vi "Image Compression with DCT.vi"() -> ()   [LabVIEW 2023]
doc: "This VI uses the DCT VI to compress images. LabVIEW transforms the Source Image to DCT Coefficients in 8-by-8 blocks, then the inverse DCT transforms the image back to Restored Image."
uses:
  <vilib>/Analysis/2dsp.llb/2D DCT.vi
  <vilib>/Analysis/2dsp.llb/2D Inverse DCT.vi
  <vilib>/Analysis/NI_AALPro.lvlib
panel:
  out "Number of block size":i32
  out "Mean Square Error (MSE)":dbl
  in  "Set All":bool
  in  "Clear All":bool
  in  "Truncated Pattern":bool[][](array[boolean])=[[TRUE, TRUE, TRUE, TRUE, FALSE, FALSE, FALSE, FALSE], [TRUE, TRUE, TRUE, FALSE, FALSE, FALSE, FALSE, FALSE], [TRUE, TRUE, FALSE, FALSE, FALSE, FALSE, FALSE, FALSE], [TRUE, FALSE, FALSE, FALSE, FALSE, FALSE, FALSE, FALSE], [FALSE, FALSE, FALSE, FALSE, FALSE, FALSE, FALSE, FALSE], [FALSE, FALSE, FALSE, FALSE, FALSE, FALSE, FALSE, FALSE], [FALSE, FALSE, FALSE, FALSE, FALSE, FALSE, FALSE, FALSE], [FALSE, FALSE, FALSE, FALSE, FALSE, FALSE, FALSE, FALSE]]
  in  "Stop":bool
  out "Restored Image":u8[][](graph)
  out "DCT Coefficients":dbl[][](graph)
  in  "Image Selector":u16(ring) items=["Cameraman", "Couple", "Columbia", "Baboon"]
  out "Source Image":u8[][](graph)
  # "Overview: Uses a Discrete Cosine Transform (DCT) to compress an image.\nRequirements: LabVIEW Full Development System\nInstructions:\n1. Run the VI and use the Image Selector to define the image to be analyzed.\n2. Modify the Truncated Pattern by clicking on the 'bits' and verify that the Mean Square Error (MSE) reduces as you enable more bits.\n3. Click Stop to stop the VI."
  # "DCT (8 X 8 block)"
  # "Inverse DCT"
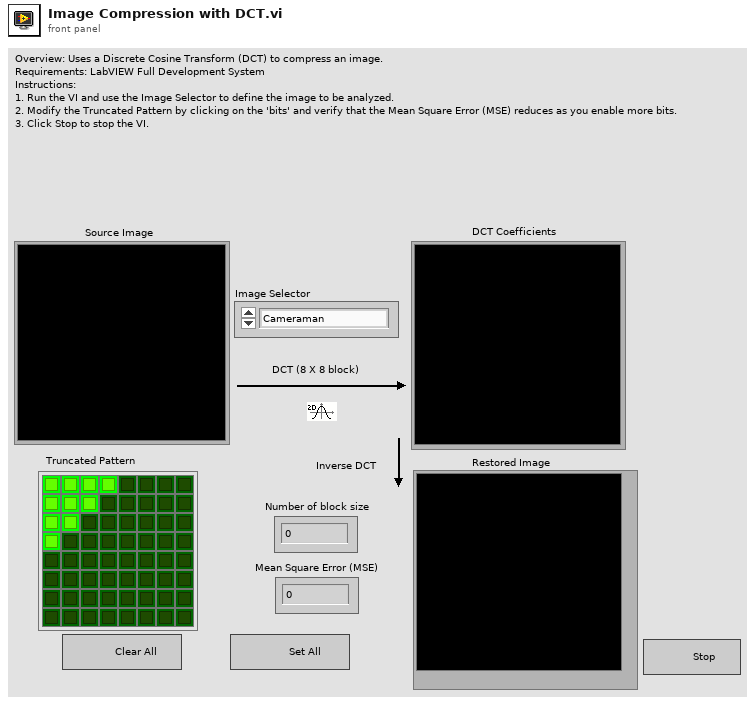
[diagram p1: front panel]
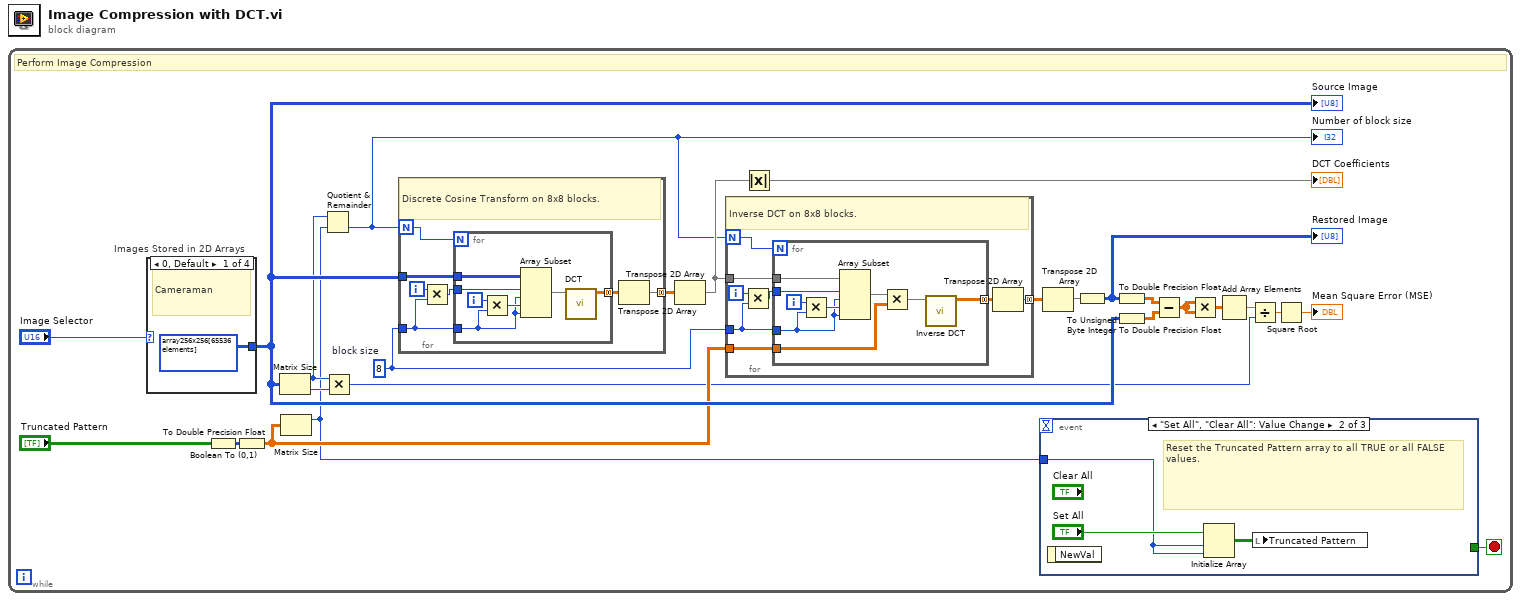
[diagram p0: block diagram]
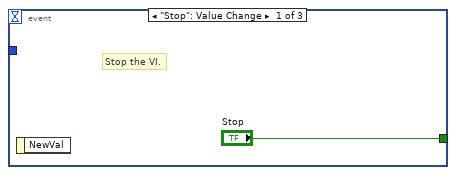
[diagram p2: hidden frame]
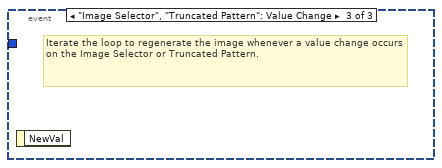
[diagram p3: hidden frame]
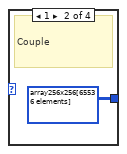
[diagram p4: hidden frame]
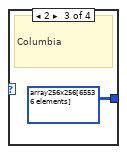
[diagram p5: hidden frame]
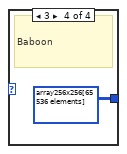
[diagram p6: hidden frame]
diagram:
  n1 = while {
    stop <- w2 stop-if-true
    w7 = 8  # block size
    # "Perform Image Compression"
    n2 = case "Images Stored in 2D Arrays" shown="0, Default" "Image Selector" {
      tunnel: [u8[][] array256x256[65536 elements] ("Image Pixels (U8)") u8[][] array256x256[65536 elements] ("Image Pixels (U8)") u8[][] array256x256[65536 elements] ("Image Pixels (U8)") u8[][] array256x256[65536 elements] ("Image Pixels (U8)")] -> w13
      frame 0, Default {
        # "Cameraman"
      }
      frame 1 {
        # "Couple"
      }
      frame 2 {
        # "Columbia"
      }
      frame 3 {
        # "Baboon"
      }
    }
    "Source Image" <- w13
    n3 = Boolean To (0,1)(Boolean="Truncated Pattern") -> (0, 1=w14:i16[][])
    n4 = To Double Precision Float(number=w14) -> (double precision float=w8:dbl[][])
    n5 = Matrix Size(0:w13) -> (1:w11:i32, 2:w12:i32)
    n6 = Matrix Size(0:w8) -> (1:w1:i32)  [unwired: 1 out]
    n7 = Quotient & Remainder(x=w11, y=w1) -> (floor(x/y)=w6:i32)  [unwired: 1 out]
    "Number of block size" <- w6
    n8 = Multiply(x=w11, y=w12) -> (x*y=w3:i32)
    n9 = for {
      N: w6 -> [w53]
      tunnel: w13 -> [w52]
      tunnel: [w50] -> w17 mode=concatenating
      tunnel: w7 -> [w48]
      i -> [w49]
      # "Discrete Cosine Transform on 8x8 blocks."
      n10 = Multiply(x=w49, y=w48) -> (x*y=w47:i32)
      n11 = for {
        N: w53 -> [_]
        tunnel: w47 -> [w60]
        tunnel: w52 -> [w59]
        tunnel: [w57] -> w51 mode=concatenating
        tunnel: w48 -> [w54]
        i -> [w55]
        n12 = Multiply(x=w55, y=w54) -> (x*y=w56:i32)
        n13 = Array Subset(array=w59, index (row)=w60, length (row)=w54, index (col)=w56, length (col)=w54) -> (w58:u8[][])
        n14 = call-poly <vilib>:"DCT.vi"("X"=w58) -> ("DCT {X}"=w57:dbl[][])  [unwired: 9 in, 1 out]
      }
      n15 = Transpose 2D Array(2D array=w51) -> (transposed array=w50:dbl[][])
    }
    n16 = Transpose 2D Array(2D array=w17) -> (transposed array=w10:dbl[][])
    n17 = for {
      N: w6 -> [w37]
      tunnel: w10 -> [w36]
      tunnel: [w34] -> w9 mode=concatenating
      tunnel: w7 -> [w32]
      tunnel: w8 -> [w30]
      i -> [w33]
      # "Inverse DCT on 8x8 blocks."
      n18 = Multiply(x=w33, y=w32) -> (x*y=w31:i32)
      n19 = for {
        N: w37 -> [_]
        tunnel: w31 -> [w46]
        tunnel: w36 -> [w45]
        tunnel: [w38] -> w35 mode=concatenating
        tunnel: w32 -> [w42]
        tunnel: w30 -> [w40]
        i -> [w43]
        n20 = Multiply(x=w43, y=w42) -> (x*y=w44:i32)
        n21 = Array Subset(array=w45, index (row)=w46, length (row)=w42, index (col)=w44, length (col)=w42) -> (w39:dbl[][])
        n22 = Multiply ("Multiply.vi")(x=w39, y=w40) -> (x*y=w41:dbl[][])
        n23 = call-poly <vilib>:"Inverse DCT.vi"("DCT {X}"=w41) -> ("X"=w38:dbl[][])  [unwired: 9 in, 1 out]
      }
      n24 = Transpose 2D Array(2D array=w35) -> (transposed array=w34:dbl[][])
    }
    n25 = Absolute Value ("Absolute Value.vi")(x=w10) -> (abs(x)=→"DCT Coefficients":dbl[][])
    n26 = event shown="[1] \"Set All\", \"Clear All\": Value Change" {
      selector: _ -> [_ _ _]
      dyn-events: _ -> [_ _ _]
      timeout: _ -> [_ _ _]
      tunnel: ["Stop" _ _] -> w2
      tunnel: w1 -> [_ w27 _]
      event "Stop": Value Change {
        # "Stop the VI."
        n27 = event-data() -> ()  [unwired: 1 in, 1 out]
      }
      event "Set All", "Clear All": Value Change {
        # "Reset the Truncated Pattern array to all TRUE or all FALSE values."
        n28 = event-data() -> ()  [unwired: 1 in, 1 out]
        n29 = Initialize Array("Set All", w27, w27) -> (w29:bool[][])
        n30 = local write "Truncated Pattern"(w29) -> ()
      }
      event "Image Selector", "Truncated Pattern": Value Change {
        # "Iterate the loop to regenerate the image whenever a value change occurs on the Image Selector or Truncated Pattern."
        n31 = event-data() -> ()  [unwired: 1 in, 1 out]
      }
    }
    n32 = Transpose 2D Array(2D array=w9) -> (transposed array=w16:dbl[][])
    n33 = To Unsigned Byte Integer(number=w16) -> (unsigned 8bit integer=w24:u8[][])
    "Restored Image" <- w24
    n34 = To Double Precision Float(number=w24) -> (double precision float=w5:dbl[][])
    n35 = To Double Precision Float(number=w13) -> (double precision float=w19:dbl[][])
    n36 = Subtract(x=w5, y=w19) -> (x-y=w4:dbl[][])
    n37 = Multiply(x=w4, y=w4) -> (x*y=w18:dbl[][])
    n38 = Add Array Elements(numeric array=w18) -> (sum=w20:dbl)
    n39 = Divide(x=w20, y=w3) -> (x/y=w21:dbl)
    n40 = Square Root(x=w21) -> (sqrt(x)=→"Mean Square Error (MSE)":dbl)
  }
